vi "Launch Tester.vi"   [LabVIEW 2020]
uses:
  Mouse/MyMouse/MyMouse.lvclass
  C:/dev/IlluminatedG/cc-maze/Maze/Mouse/Mouse.lvclass
  App/MazeUI/MazeUI.lvclass
panel:
  # "Run this VI to load the Maze App with your mouse implementation.\n\nYou will need to close the Maze App UI to edit your implementation again."
types:
  T1 = enum32{"Invalid", "Standard", "Closed", "Hidden", "Minimized", "Maximized"}
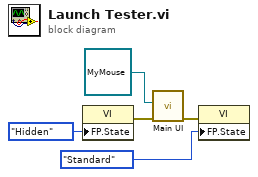
[diagram p0: block diagram]
diagram:
  n1 = property class="VI"("FP.State"=T1."Hidden" ("Front Panel Window:State")) -> (error out=w4:errorcluster)  [unwired: 2 in, 1 out]
  n2 = call "Main UI.vi"("error in (no error)"=w4, "Initial Mouse (Demo)"=refnum<class "MyMouse.lvclass"> refnum ("Mouse.lvlib:MyMouse.lvclass")) -> ("error out"=w1:errorcluster)  [unwired: 9 in]
  n3 = property class="VI"(error in=w1, "FP.State"=T1."Standard" ("Front Panel Window:State")) -> ()  [unwired: 1 in, 2 out]
